vi "ImplicitParameterNode_Create.vi"(0 "reference":refnum<class "ImplicitParameterNode.lvclass">, 5 "error in (no error)":errorcluster, 6 "GoopReferenceIn":T1) -> (14 "reference out":refnum<class "ImplicitParameterNode.lvclass">, 16 "# of objects":i32, 19 "error out":errorcluster)   [LabVIEW 2014, in "ImplicitParameterNode.lvclass"]
doc: "Creates and initializes a new ImplicitParameterNode object.\n\nThis object should be destroyed using a ImplicitParameterNode destructor VI or a virtual base class destructor VI.\n\n[GOOP 2.3]"
uses:
  <resource>/Framework/Providers/Open_GDS/UML/ImplicitParameterNode_class/ImplicitParameterNode.lvclass
  <resource>/Framework/Providers/Open_GDS/UML/AbstractNode_class/ObjectReference.ctl
  <resource>/Framework/Providers/Open_GDS/UML/General/Rectangle/Rectangle Rectangle2D.ctl
  <resource>/Framework/Providers/Open_GDS/UML/RectangularNode_class/RectangularNode.lvclass
  <resource>/Framework/Providers/Open_GDS/UML/MultiLineString_class/MultiLineString.lvclass
  <resource>/Framework/Providers/Open_GDS/UML/AbstractNode_class/AbstractNode.lvclass
panel:
  # "The input reference should only\nbe wired when this method is called\nby a sub class constructor."
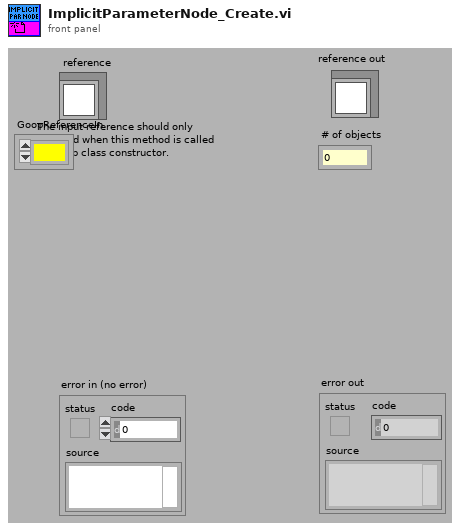
[diagram p1: front panel]
types:
  T1 = typedef "AbstractNode.lvclass/ObjectReference.ctl" = refnum<k1>
  T2 = typedef "Rectangle Rectangle2D.ctl" = cluster{"x":dbl, "y":dbl, "width":dbl, "height":dbl}
  T3 = typedef "ImplicitParameterNode.lvclass/ObjectAttributes.ctl" = cluster{"Base class":T4, "topHeight":dbl, "name":refnum<class "MultiLineString.lvclass">, "DEFAULT_TOP_HEIGHT":i32, "DEFAULT_WIDTH":i32, "DEFAULT_HEIGHT":i32}
  T4 = typedef "RectangularNode.lvclass/ObjectAttributes.ctl" = cluster{"Base class":T5, "bounds":T2}
  T5 = typedef "AbstractNode.lvclass/ObjectAttributes.ctl" = cluster{"parent":refnum<class "AbstractNode.lvclass">, "children":refnum<class "AbstractNode.lvclass">[], "Hidden":bool}
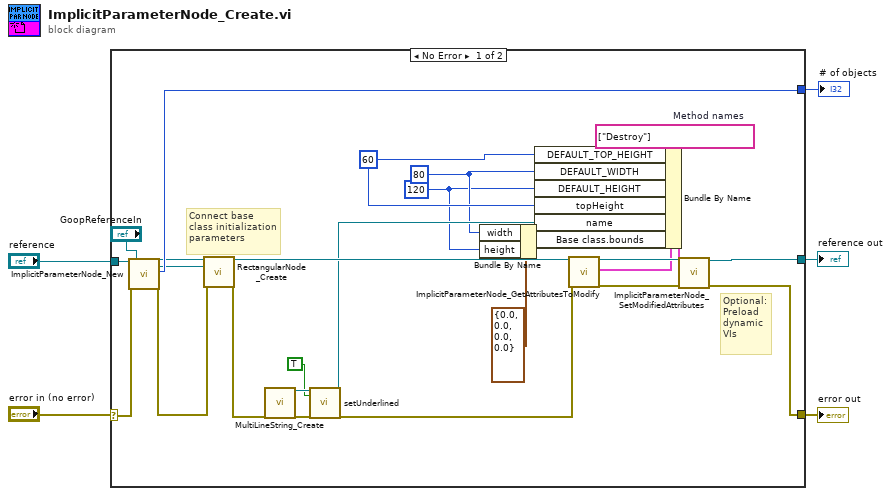
[diagram p0: block diagram]
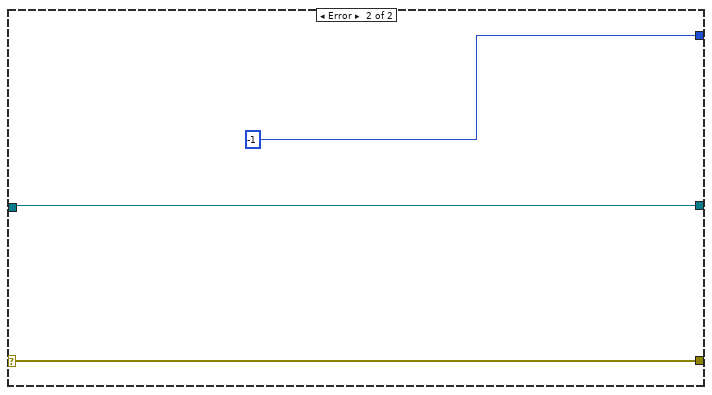
[diagram p2: hidden frame]
diagram:
  n1 = case shown="No Error" "error in (no error)" {
    selector: "error in (no error)" -> [w30 w32]
    tunnel: [w20 w31] -> w5
    tunnel: [w19 w32] -> w4
    tunnel: [w29 -1 ("Nr of open handles")] -> w3
    tunnel: "reference" -> [w28 w31]
    frame No Error {
      (unwired) string[] ["Destroy"]  # Method names
      w8 = 120 ("DEFAULT_HEIGHT")
      w9 = 80 ("DEFAULT_WIDTH")
      w18 = 60 ("DEFAULT_TOP_HEIGHT")
      # "Optional:\nPreload\ndynamic\nVIs"
      # "Connect base\nclass initialization\nparameters"
      n2 = call <resource>:"ImplicitParameterNode_New.vi"("reference in"=w28, "error in (no error)"=w30, "GoopReferenceIn"="GoopReferenceIn") -> ("GoopReferenceOut"=w6:T1, "reference out"=w25:refnum<class "ImplicitParameterNode.lvclass">, "# of objects"=w29:i32, "error out"=w27:errorcluster)  [unwired: 2 in, 11 out]
      n3 = call <resource>:"RectangularNode_Create.vi"("reference"=w25, "error in (no error)"=w27, "GoopReferenceIn"=w6) -> ("reference out"=w24:refnum<class "ImplicitParameterNode.lvclass">, "error out"=w17:errorcluster)  [unwired: 15 out]
      n4 = call <resource>:"MultiLineString_Create.vi"("error in (no error)"=w17) -> ("reference out"=w16:refnum<class "MultiLineString.lvclass">, "error out"=w15:errorcluster)  [unwired: 3 in, 14 out]
      n5 = call <resource>:"setUnderlined.vi"("reference"=w16, "underlined"=TRUE, "error in (no error)"=w15) -> ("reference out"=w13:refnum<class "MultiLineString.lvclass">, "error out"=w12:errorcluster)  [unwired: 15 out]
      n6 = Bundle By Name(cluster=T2 {"x"=0.0, "y"=0.0, "width"=0.0, "height"=0.0} ("Base class.bounds"), "width"=w9, "height"=w8) -> (w10:T2)
      n7 = call <resource>:"ImplicitParameterNode_GetAttributesToModify.vi"("reference in"=w24, "error in (no error)"=w12) -> ("reference out"=w23:refnum<class "ImplicitParameterNode.lvclass">, "Attributes"=w22:T3, "error out"=w26:errorcluster)  [unwired: 1 in, 14 out]
      n8 = Bundle By Name(cluster=w22, "DEFAULT_TOP_HEIGHT"=w18, "DEFAULT_WIDTH"=w9, "DEFAULT_HEIGHT"=w8, "topHeight"=w18, "name"=w13, "Base class.bounds"=w10) -> (w21:T3)
      n9 = call <resource>:"ImplicitParameterNode_SetModifiedAttributes.vi"("reference in"=w23, "Attributes"=w21, "error in (no error)"=w26) -> ("reference out"=w20:refnum<class "ImplicitParameterNode.lvclass">, "error out"=w19:errorcluster)  [unwired: 3 in, 12 out]
    }
    frame Error {
    }
  }
  "error out" <- w4
  "reference out" <- w5
  "# of objects" <- w3
